vi "addEdge.vi"(0 "reference":refnum<class "ImplicitParameterNode.lvclass">, 1 "egde":refnum<class "AbstractEdge.lvclass">, 2 "p1":T1 {"y" format="%.2f"; "x" format="%.2f"}, 3 "p2":T1 {"y" format="%.2f"; "x" format="%.2f"}, 5 "error in (no error)":errorcluster) -> (14 "reference out":refnum<class "ImplicitParameterNode.lvclass">, 15 "add":bool, 19 "error out":errorcluster)   [LabVIEW 2016, in "ImplicitParameterNode.lvclass"]
doc: "public boolean addEdge(Edge e, Point2D p1, Point2D p2)"
uses:
  <resource>/Framework/Providers/Open_GDS/UML/ImplicitParameterNode_class/ImplicitParameterNode.lvclass
  <resource>/Framework/Providers/Open_GDS/UML/AbstractEdge_class/AbstractEdge.lvclass
  <resource>/Framework/Providers/Open_GDS/UML/General/Point/Point Point2D.ctl
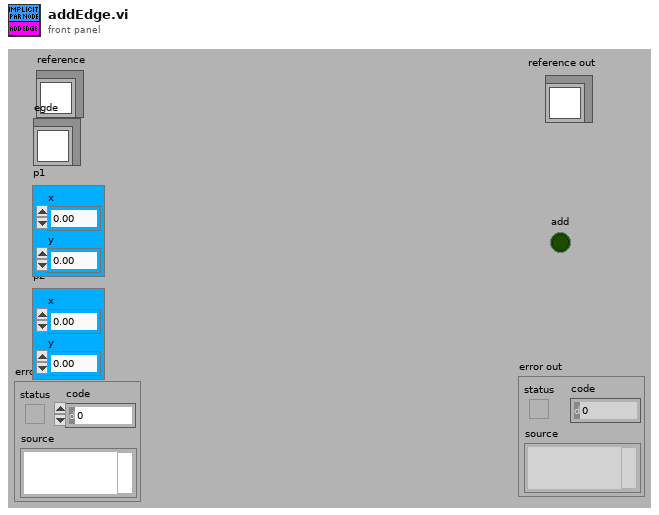
[diagram p1: front panel]
types:
  T1 = typedef "Point Point2D.ctl" = cluster{"x":dbl, "y":dbl}
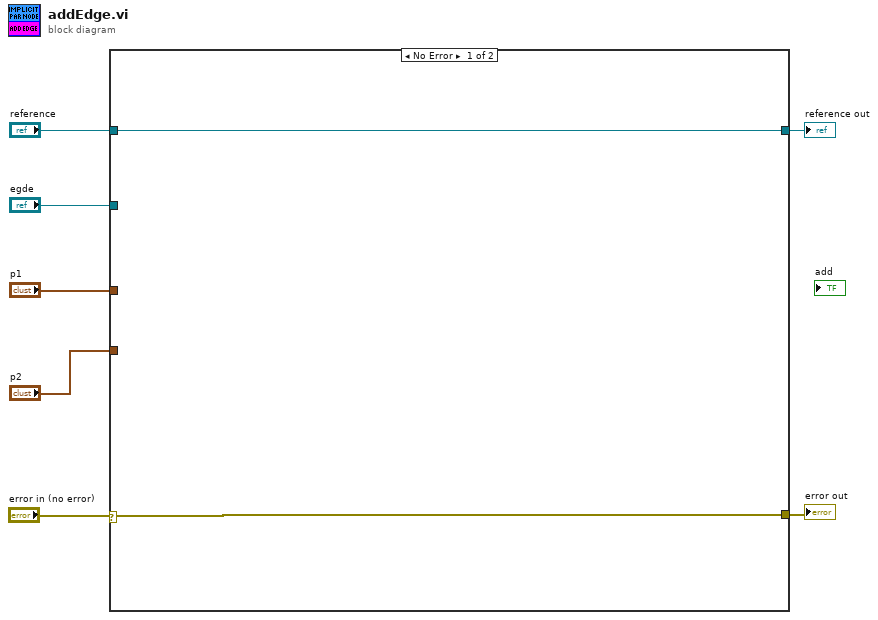
[diagram p0: block diagram]
diagram:
  n1 = case shown="No Error" "error in (no error)" {
    selector: "error in (no error)" -> [w8 w10]
    tunnel: "reference" -> [w9 w11]
    tunnel: [w8 w10] -> w6
    tunnel: [w9 w11] -> w5
    tunnel: "egde" -> [_ _]
    tunnel: "p1" -> [_ _]
    tunnel: "p2" -> [_ _]
    frame No Error {
    }
    frame Error {
    }
  }
  "reference out" <- w5
  "error out" <- w6
